vi "温室大棚.vi"() -> ()   [LabVIEW 2018]
panel:
  out "报警指示灯":bool
  out "状态显示":string
  out "当前温度":dbl(slide) scale=0.0..100.0
  in  "温度下限":dbl
  in  "温度上限":dbl
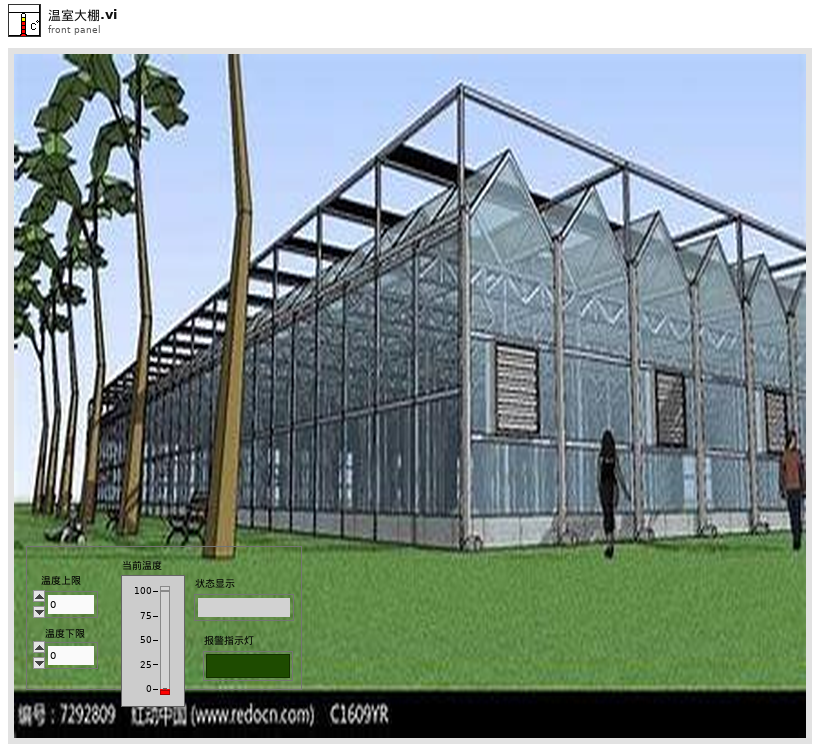
[diagram p1: front panel]
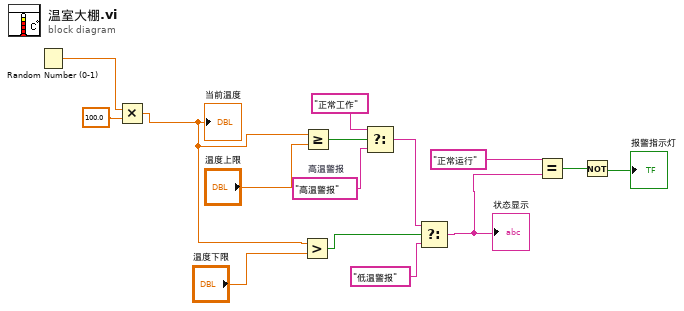
[diagram p0: block diagram]
diagram:
  w6 = "高温警报"  # 高温警报
  n1 = Random Number (0-1)() -> (number: 0 to 1=w14:dbl)
  n2 = Multiply(x=w14, y=100.0) -> (x*y=w10:dbl)
  "当前温度" <- w10
  n3 = Greater?(x=w10, y="温度下限") -> (0:w8:bool)
  n4 = Greater Or Equal?(x=w10, y="温度上限") -> (x >= y?=w12:bool)
  n5 = Select(t="正常工作", s=w12, f=w6) -> (s? t:f=w7:string)
  n6 = Select(t=w7, s=w8, f="低温警报") -> (s? t:f=w3:string)
  "状态显示" <- w3
  n7 = Equal?(x="正常运行", y=w3) -> (x = y?=w2:bool)
  n8 = Not(x=w2) -> (.not. x?=→"报警指示灯":bool)
